vi "DirettoreClose.vi"(11 "FPGAReference":refnum<k20>) -> (0 "ErrorOut":errorcluster)   [LabVIEW 2012]
uses:
  <vilib>/FPGAPlugInAG/Dynamic/niLvFpga_Close_Dynamic.vi
  <vilib>/rvi/interface/nirviCloseFPGA/nirviCloseFPGA.xnode
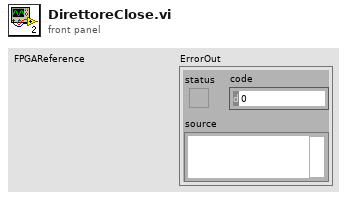
[diagram p1: front panel]
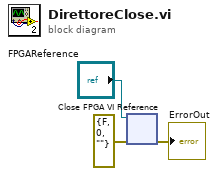
[diagram p0: block diagram]
diagram:
  n1 = xnode "Close FPGA VI Reference"("FPGA VI Reference In"="FPGAReference", "error in"=errorcluster {"status"=FALSE, "code"=0, "source"=""}) -> ("error out"=→"ErrorOut":errorcluster)
